vi "Delete Destination Tags.vi"(8 "error in (no error)":errorcluster, 11 "BuildSpec in":refnum<vi>) -> (0 "error out":errorcluster, 3 "BuildSpec out":refnum<vi>)   [LabVIEW 2019, in "Project Sync Tools.lvclass"]
uses:
  Project Sync Tools.lvclass
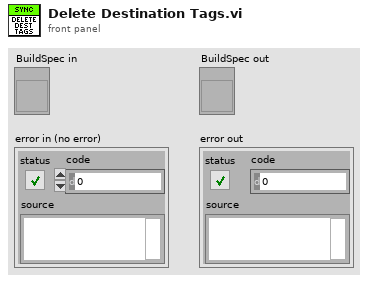
[diagram p1: front panel]
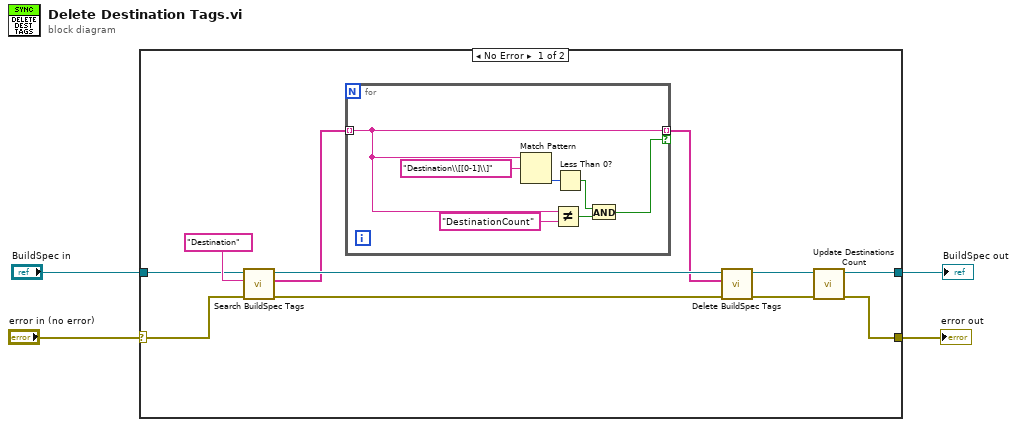
[diagram p0: block diagram]
diagram:
  n1 = case shown="No Error" "error in (no error)" {
    selector: "error in (no error)" -> [w5 w23]
    tunnel: "BuildSpec in" -> [w14 w24]
    tunnel: [w7 w24] -> w3
    tunnel: [w6 w23] -> w2
    frame No Error {
      n2 = call "Search BuildSpec Tags.vi"("error in (no error)"=w5, "Regular expression"="Destination", "BuildSpec in"=w14) -> ("error out"=w13:errorcluster, "Tag Names"=w11:string[], "BuildSpec out"=w12:refnum<vi>)  [unwired: 6 in]
      n3 = for {
        tunnel: w11 -> [w19] mode=indexing
        tunnel: [w19] -> w10 mode=indexing if=w16
        n4 = Match Pattern(string=w19, regular expression="Destination\\[[0-1]\\]") -> (offset past match=w21:i32)  [unwired: 1 in, 3 out]
        n5 = Not Equal?(x=w19, y="DestinationCount" ("regular expression")) -> (x != y?=w18:bool)
        n6 = Less Than 0?(x=w21) -> (x < 0?=w17:bool)
        n7 = And(x=w17, y=w18) -> (x .and. y?=w16:bool)
      }
      n8 = call "Delete BuildSpec Tags.vi"("error in (no error)"=w13, "Tag Names"=w10, "ProjectItem in"=w12) -> ("error out"=w9:errorcluster, "ProjectItem out"=w8:refnum<vi>)  [unwired: 6 in, 1 out]
      n9 = call "Update Destinations Count.vi"("error in (no error)"=w9, "BuildSpec in"=w8) -> ("error out"=w6:errorcluster, "BuildSpec out"=w7:refnum<vi>)  [unwired: 8 in]
    }
    frame Error {
    }
  }
  "BuildSpec out" <- w3
  "error out" <- w2
